vi "Smart laser Pointer.vi"(8 "Y pos":dbl=166.0, 9 "X Pos":dbl=170.0, 10 "Y Parameters":T1={"Number of Y Steps"=200, "Max Y (V)"=1.0, "Min Y (V)"=-1.0}, 11 "X Parameters":T2={"Number of X Steps"=200, "Max X (V)"=1.0, "Min X (V)"=-1.0}) -> ()   [LabVIEW 2011]
uses:
  <vilib>/DAQmx/write.llb/DAQmx Write (Analog 2D DBL NChan NSamp).vi
  <vilib>/DAQmx/create/channels.llb/DAQmx Create Channel (AO-Voltage-Basic).vi
  <vilib>/DAQmx/miscellaneous.llb/DAQmx Fill In Error Info.vi
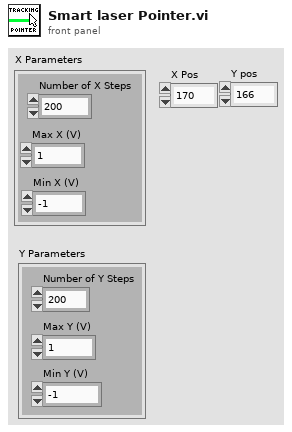
[diagram p1: front panel]
types:
  T1 = cluster{"Number of Y Steps":i32, "Max Y (V)":dbl, "Min Y (V)":dbl}
  T2 = cluster{"Number of X Steps":i32, "Max X (V)":dbl, "Min X (V)":dbl}
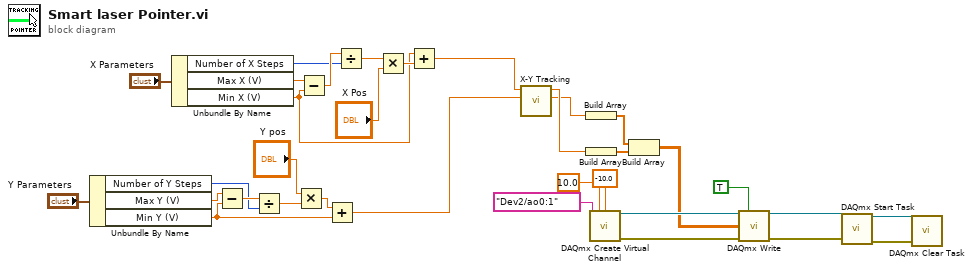
[diagram p0: block diagram]
diagram:
  n1 = Unbundle By Name("Y Parameters") -> ("Number of Y Steps"=w25:i32, "Max Y (V)"=w24:dbl, "Min Y (V)"=w23:dbl)
  n2 = Unbundle By Name("X Parameters") -> ("Number of X Steps"=w21:i32, "Max X (V)"=w20:dbl, "Min X (V)"=w19:dbl)
  n3 = Subtract(x=w24, y=w23) -> (x-y=w33:dbl)
  n4 = Divide(x=w33, y=w25) -> (x/y=w30:dbl)
  n5 = Multiply(x="Y pos", y=w30) -> (x*y=w29:dbl)
  n6 = Subtract(x=w20, y=w19) -> (x-y=w32:dbl)
  n7 = Add(x=w29, y=w23) -> (x+y=w1:dbl)
  n8 = Divide(x=w32, y=w21) -> (x/y=w27:dbl)
  n9 = Multiply(x=w27, y="X Pos") -> (x*y=w26:dbl)
  n10 = Add(x=w19, y=w26) -> (x+y=w2:dbl)
  n11 = call "X-Y Tracking.vi"("Y Voltage"=w1, "X Voltage"=w2) -> ("Y centered Voltage"=w3:dbl, "X Centered Voltage"=w4:dbl)  [unwired: 3 in, 5 out]
  n12 = Build Array(w3) -> (w7:dbl[])
  n13 = Build Array(w4) -> (w6:dbl[])
  n14 = call-poly <vilib>:"DAQmx Create Virtual Channel.vi"("maximum value"=10.0, "minimum value"=-10.0, "physical channels"=tag "Dev2/ao0:1") -> ("task out"=w14:refnum<k21>, "error out"=w13:errorcluster)  [unwired: 11 in]
  n15 = Build Array(w7, w6) -> (w5:dbl[][])
  n16 = call-poly <vilib>:"DAQmx Write.vi"("task/channels in"=w14, "auto start"=TRUE, "data"=w5, "error in"=w13) -> ("task out"=w12:refnum<k21>, "error out"=w11:errorcluster)  [unwired: 9 in, 1 out]
  n17 = call <vilib>:"DAQmx Start Task.vi"("task/channels in"=w12, "error in"=w11) -> ("task out"=w10:refnum<k21>, "error out"=w9:errorcluster)  [unwired: 12 in]
  n18 = call <vilib>:"DAQmx Clear Task.vi"("task in"=w10, "error in"=w9) -> ()  [unwired: 13 in, 1 out]
